vi "maxificator.vi"(6 "first time":bool=TRUE, 7 "size":i32=1, 11 "number":dbl) -> (2 "max":dbl)   [LabVIEW 2010]
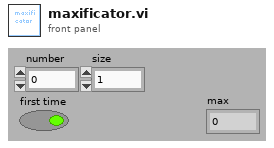
[diagram p1: front panel]
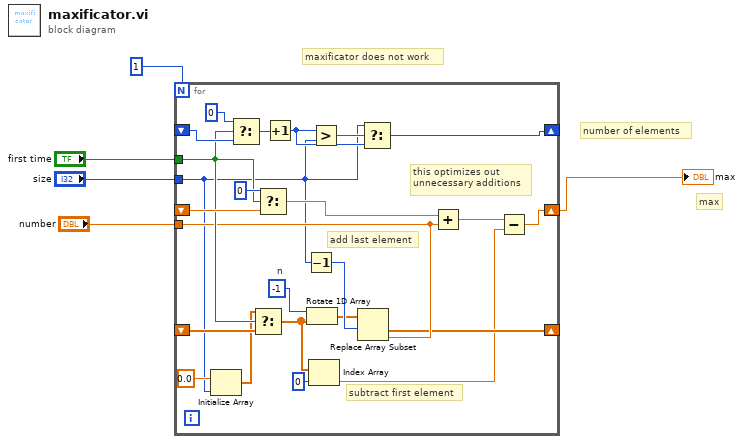
[diagram p0: block diagram]
diagram:
  # "maxificator does not work"
  # "max"
  # "number of elements"
  n1 = for {
    N: 1 -> [_]
    tunnel: "first time" -> [w20]
    shift-right: [w12] -> w1
    shift-left: _ -> [w24]
    shift-right: [w26] -> _
    shift-left: _ -> [w28]
    tunnel: "size" -> [w6]
    tunnel: "number" -> [w17]
    shift-right: [w14] -> _
    shift-left: _ -> [w19]
    w18 = -1  # n
    # "add last element"
    # "subtract first element"
    # "this optimizes out \nunnecessary additions"
    n2 = Initialize Array(0.0, w6) -> (w7:dbl[])
    n3 = Select(t=0, s=w20, f=w28) -> (s? t:f=w22:i32)
    n4 = Select(t=w7, s=w20, f=w19) -> (s? t:f=w10:dbl[])
    n5 = Select(t=0, s=w20, f=w24) -> (s? t:f=w23:dbl)
    n6 = Increment(x=w22) -> (x+1=w21:i32)
    n7 = Decrement(x=w6) -> (x-1=w16:i32)
    n8 = Rotate 1D Array(1:w10, 2:w18) -> (0:w15:dbl[])
    n9 = Index Array(array=w10, index=0) -> (element=w9:dbl)
    n10 = Greater?(x=w21, y=w6) -> (0:w27:bool)
    n11 = Replace Array Subset(array=w15, new element=w17, index=w16) -> (w14:dbl[])
    n12 = Select(t=w6, s=w27, f=w21) -> (s? t:f=w26:i32)
    n13 = Add(x=w23, y=w17) -> (x+y=w13:dbl)
    n14 = Subtract(x=w13, y=w9) -> (x-y=w12:dbl)
  }
  "max" <- w1
